vi "BotSpeak.TestCom.vi"(2 "Termination":string="\r\n", 3 "Bot Settings":T1) -> (0 "firmware":dbl, 1 "Bot Settings out":T1)   [LabVIEW 2012]
uses:
  <userlib>/BotSpeak/VIs/Direct/BotSpeak_Control.ctl
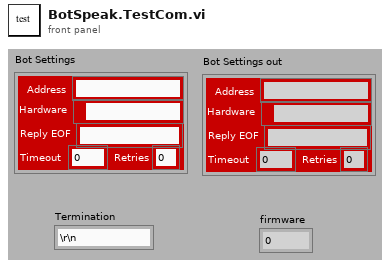
[diagram p1: front panel]
types:
  T1 = typedef "BotSpeak_Control.ctl" = cluster{"Address":string, "Reply EOF":string, "Hardware":path, "Retries":i8, "Timeout":i32}
  T2 = typedef "CommState.ctl" = cluster{"Bot Settings":T1, "Initialized":bool, "Talking":bool}
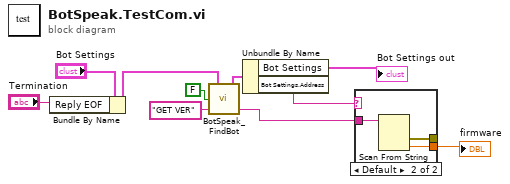
[diagram p0: block diagram]
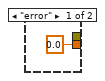
[diagram p2: hidden frame]
diagram:
  n1 = Bundle By Name(cluster="Bot Settings", "Reply EOF"="Termination") -> (w6:T1)
  n2 = call <userlib>:"BotSpeak_FindBot.vi"("String To Send"="GET VER" ("URAPI"), "Reset?"=FALSE, "Bot Settings"=w6) -> ("Reply"=w1:string, "Connection"=w5:T2)  [unwired: 1 out]
  n3 = Unbundle By Name(w5) -> ("Bot Settings"=→"Bot Settings out":T1, "Bot Settings.Address"=w2:string)
  n4 = case shown="Default" w2 {
    tunnel: [0.0 w14] -> w10
    tunnel: w1 -> [_ w13]
    tunnel: [_ w12] -> _
    frame "error" {
    }
    frame Default {
      n5 = Scan From String(input string=w13) -> (error out=w12:errorcluster, output 1=w14:dbl)  [unwired: 4 in, 2 out]
    }
  }
  "firmware" <- w10
